vi "Motor State.vi"() -> ()   [LabVIEW 2017]
uses:
  Motor State.ctl
panel:
  out "Motor State 2":T1
  out "Motor State":T1
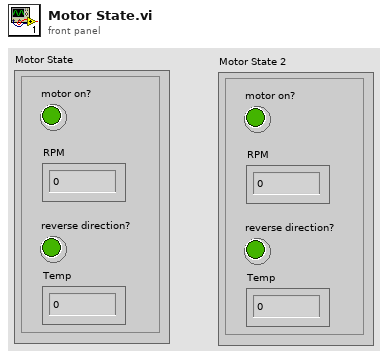
[diagram p1: front panel]
types:
  T1 = typedef "Motor State.ctl" = cluster{"motor on?":bool, "RPM":dbl, "reverse direction?":bool, "Temp":dbl}
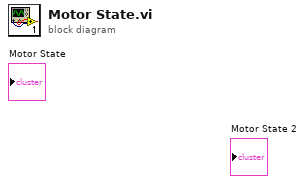
[diagram p0: block diagram]
diagram:
